vi "BRig_RT__Case_Exp__endTrial_checkFreeReward__v17.vi"(6 "input_dataBlock":u16[][](array[numeric]), 8 "input_dataExp":u16[](array[numeric]), 9 "input_dataTrial":u16[][](array[numeric]), 10 "input_dataCurrent":u16[](array[numeric])) -> (3 "output_state":T1, 5 "output_endBlock":bool)   [LabVIEW 2014]
uses:
  myRIO_BRig_RT__Case_Exp_stateList.ctl
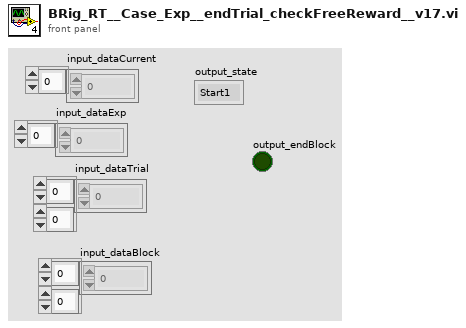
[diagram p1: front panel]
types:
  T1 = typedef "myRIO_BRig_RT__Case_Exp_stateList.ctl" = enum16{"Start1", "Start2", "Start3", "saveSettings1", "saveSettings2", "saveSettings3", "saveSettings4", "saveSettings_LC_ENL_l1", "saveSettings_LC_ENL_l2", "saveSettings_LC_Cue_l1", "saveSettings_LC_Cue_l2", "saveSettings6_LC_l1_Other", "SaveSettings6_LC_l2_Other", "setSettings_Audio", "setSettings_Laser", "initBlock_pre", "initBlock", "initBlock2", "initBlock_post", "initTrial_pre", "initTrial", "initTrial2", "initTrial3", "initTrial4", "initTrial_LC_ENL1", "initTrial_LC_Cue1", "initTrial_LC_Cue1_2", "initTrial_LC_Sel", "initTrial_post", "ENL1_pre", "ENL1", "ENL1_post", "ENL1Penalty_pre", "ENL1Penalty", "ENL2_pre", "ENL2", "ENL2Penalty_pre", "ENL2Penalty", "Cue1_pre", "Cue1", "Cue1_post", "Cue1Penalty_pre", "Cue1Penalty", "Cue2_pre", "Cue2", "Cue2Penalty_pre", "Cue2Penalty", "Selection_pre", "Selection", "Select_post", "SelectReward_pre", "SelectReward", "SelectRewardPost_pre", "SelectRewardPost", "SelectWrong_pre", "SelectWrong", "SelectWrong_post", "SelectTimeout_pre", "SelectTimeout", "SelectTimeout_post", "endTrial_pre", "endTrial1", "endTrial2", "endTrial3", "endTrial_post", "endBlock_pre", "endBlock", "endBlock_post", "endExp", "commConnect", "commUpload_pre", "commUpload_dataBlock", "commUpload_dataCurrent", "commUpload_dataExp", "commUpload_dataLC", "commUpload_dataTrial", "commUpload_post", "saveData_pre", "saveData_dataBlock", "saveData_dataCurrent", "saveData_dataExp", "saveData_dataLC", "saveData_dataTrial", "saveData_post", "empty_endBlock1", "empty_endBlock2", "empty_endTrial1", "empty_endTrial2", "empty_endTrial3", "empty_endTrial4", "empty_endTrial5", "dummyState", "dummyState_endBlock", "FreeReward_pre", "FreeReward", "FreeRewardPost_pre", "FreeRewardPost"}
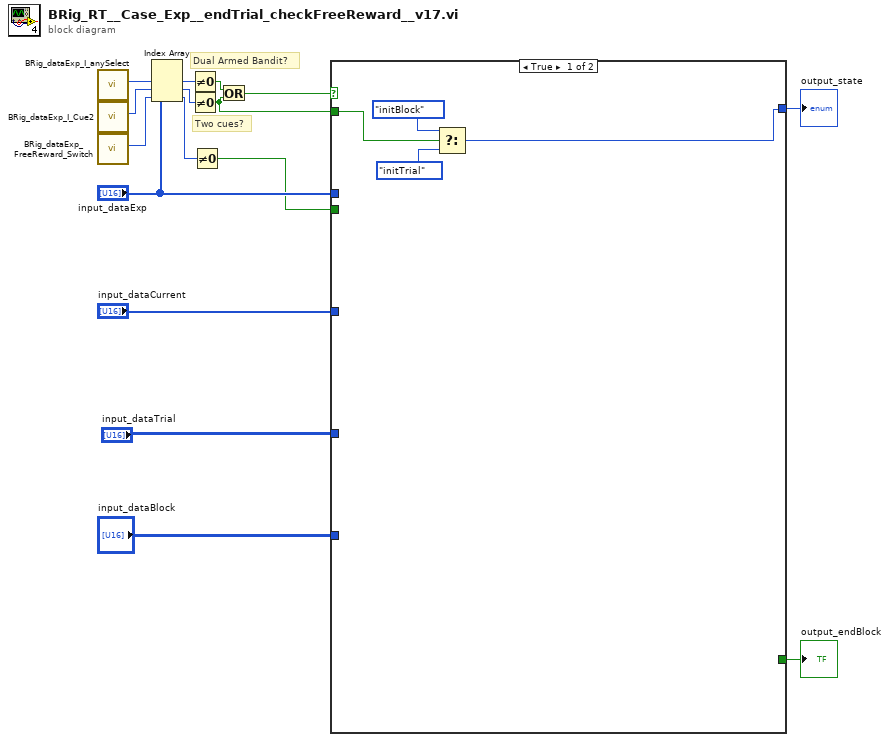
[diagram p0: block diagram]
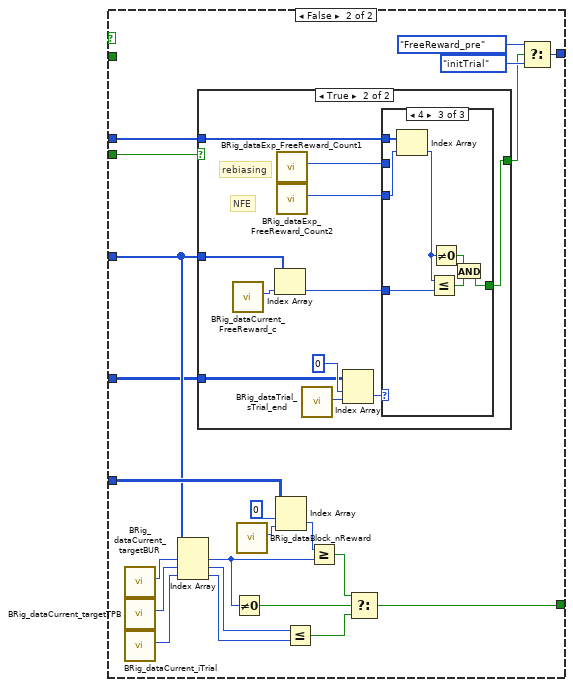
[diagram p2: hidden frame]
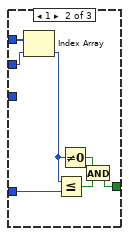
[diagram p5: hidden frame]
diagram:
  # "Two cues?"
  # "Dual Armed Bandit?"
  n1 = call "BRig_dataExp_I_anySelect.vi"() -> ("output_I_anySelect"=w11:i32)  [unwired: 11 in]
  n2 = call "BRig_dataExp_I_Cue2.vi"() -> ("output_I_Cue2"=w9:i32)  [unwired: 11 in]
  n3 = call "BRig_dataExp_FreeReward_Switch.vi"() -> ("output_FreeReward_Switch"=w3:i32)  [unwired: 11 in]
  n4 = Index Array(array="input_dataExp", index #1=w11, index #2=w9, index #3=w3) -> (element #1=w10:u16, element #2=w8:u16, element #3=w2:u16)
  n5 = Not Equal To 0?(x=w10) -> (x != 0?=w7:bool)
  n6 = Not Equal To 0?(x=w8) -> (x != 0?=w5:bool)
  n7 = Not Equal To 0?(x=w2) -> (x != 0?=w1:bool)
  n8 = Or(x=w7, y=w5) -> (x .or. y?=w6:bool)
  n9 = case shown="True" w6 {
    tunnel: w1 -> [_ w40]
    tunnel: "input_dataExp" -> [_ w39]
    tunnel: [w18 w37] -> w16
    tunnel: [_ w35] -> w15
    tunnel: "input_dataBlock" -> [_ w30]
    tunnel: "input_dataCurrent" -> [_ w22]
    tunnel: "input_dataTrial" -> [_ w21]
    tunnel: w5 -> [w20 _]
    frame True {
      n10 = Select(t=myRIO_BRig_RT__Case_Exp_stateList."initBlock", s=w20, f=myRIO_BRig_RT__Case_Exp_stateList."initTrial" ("Enum")) -> (s? t:f=w18:T1)
    }
    frame False {
      n11 = call "BRig_dataCurrent_targetBUR.vi"() -> ("output_targetBUR"=w24:i32)  [unwired: 11 in]
      n12 = call "BRig_dataCurrent_targetTPB.vi"() -> ("output_targetTPB"=w23:i32)  [unwired: 11 in]
      n13 = call "BRig_dataCurrent_iTrial.vi"() -> ("output_iTrial"=w25:i32)  [unwired: 11 in]
      n14 = Index Array(array=w22, index #1=w24, index #2=w23, index #3=w25) -> (element #1=w33:u16, element #2=w26:u16, element #3=w27:u16)
      n15 = case shown="True" w40 {
        selector: w40 -> [w43 _]
        tunnel: w39 -> [_ w51]
        tunnel: [w43 w47] -> w38
        tunnel: w22 -> [_ w45]
        tunnel: w21 -> [_ w44]
        frame False {
        }
        frame True {
          # "NFE"
          # "rebiasing"
          n16 = call "BRig_dataCurrent_FreeReward_c.vi"() -> ("output_FreeReward_c"=w54:i32)  [unwired: 11 in]
          n17 = Index Array(array=w45, index=w54) -> (element=w48:u16)
          n18 = call "BRig_dataExp_FreeReward_Count1.vi"() -> ("output_FreeReward_Count"=w50:i32)  [unwired: 11 in]
          n19 = call "BRig_dataExp_FreeReward_Count2.vi"() -> ("output_FreeReward_Count"=w49:i32)  [unwired: 11 in]
          n20 = call "BRig_dataTrial_sTrial_end.vi"() -> ("output_sTrial_end"=w53:i32)  [unwired: 11 in]
          n21 = Index Array(array=w44, index (row)=0, index (col)=w53) -> (element=w52:u16)
          n22 = case shown="4" w52 {
            tunnel: w51 -> [_ w61 w68]
            tunnel: w50 -> [_ w60 _]
            tunnel: w49 -> [_ _ w66]
            tunnel: w48 -> [_ w59 w67]
            tunnel: [_ w55 w62] -> w47
            frame 0, Default {
            }
            frame 1 {
              n23 = Index Array(array=w61, index=w60) -> (element=w58:u16)
              n24 = Less Or Equal?(x=w58, y=w59) -> (x <= y?=w57:bool)
              n25 = Not Equal To 0?(x=w58) -> (x != 0?=w56:bool)
              n26 = And(x=w56, y=w57) -> (x .and. y?=w55:bool)
            }
            frame 4 {
              n27 = Index Array(array=w68, index=w66) -> (element=w64:u16)
              n28 = Less Or Equal?(x=w64, y=w67) -> (x <= y?=w63:bool)
              n29 = Not Equal To 0?(x=w64) -> (x != 0?=w65:bool)
              n30 = And(x=w65, y=w63) -> (x .and. y?=w62:bool)
            }
          }
        }
      }
      n31 = Not Equal To 0?(x=w33) -> (x != 0?=w28:bool)
      n32 = call "BRig_dataBlock_nReward.vi"() -> ("output_nReward"=w31:i32)  [unwired: 11 in]
      n33 = Index Array(array=w30, index (row)=0, index (col)=w31) -> (element=w32:u16)
      n34 = Less Or Equal?(x=w26, y=w27) -> (x <= y?=w29:bool)
      n35 = Greater Or Equal?(x=w32, y=w33) -> (x >= y?=w34:bool)
      n36 = Select(t=w34, s=w28, f=w29) -> (s? t:f=w35:bool)
      n37 = Select(t=myRIO_BRig_RT__Case_Exp_stateList."FreeReward_pre" ("Enum"), s=w38, f=myRIO_BRig_RT__Case_Exp_stateList."initTrial" ("Enum")) -> (s? t:f=w37:T1)
    }
  }
  "output_state" <- w16
  "output_endBlock" <- w15
